vi "Handle Import.vi"(4 "Search Paths":path[](array[path]), 6 "Source .proto":path, 7 "Enumerations in":map{string, T1}(c390), 8 "error in (no error)":errorcluster, 9 "Messages in":map{string, T3}(c390), 10 "Import String":string, 11 "ProtoParser in":refnum<class "ProtoParser.lvclass">) -> (0 "error out":errorcluster, 1 "Messages":map{string, T3}(c390), 3 "ProtoParser out":refnum<class "ProtoParser.lvclass">, 5 "Enumerations":map{string, T1}(c390))   [LabVIEW 2020, in "LV-Protoc.lvlib" / "ProtoParser.lvclass"]
uses:
  ProtoParser.lvclass
  LV-Proto/Message.ctl
  LV-Proto/Field.ctl
  LV-Proto/Type.ctl
  LV-Proto/Proto Type.ctl
  LV-Proto/Enumeration.ctl
  LV-Proto/Enum Value.ctl
  LV-Proto/LV-Proto.lvlib
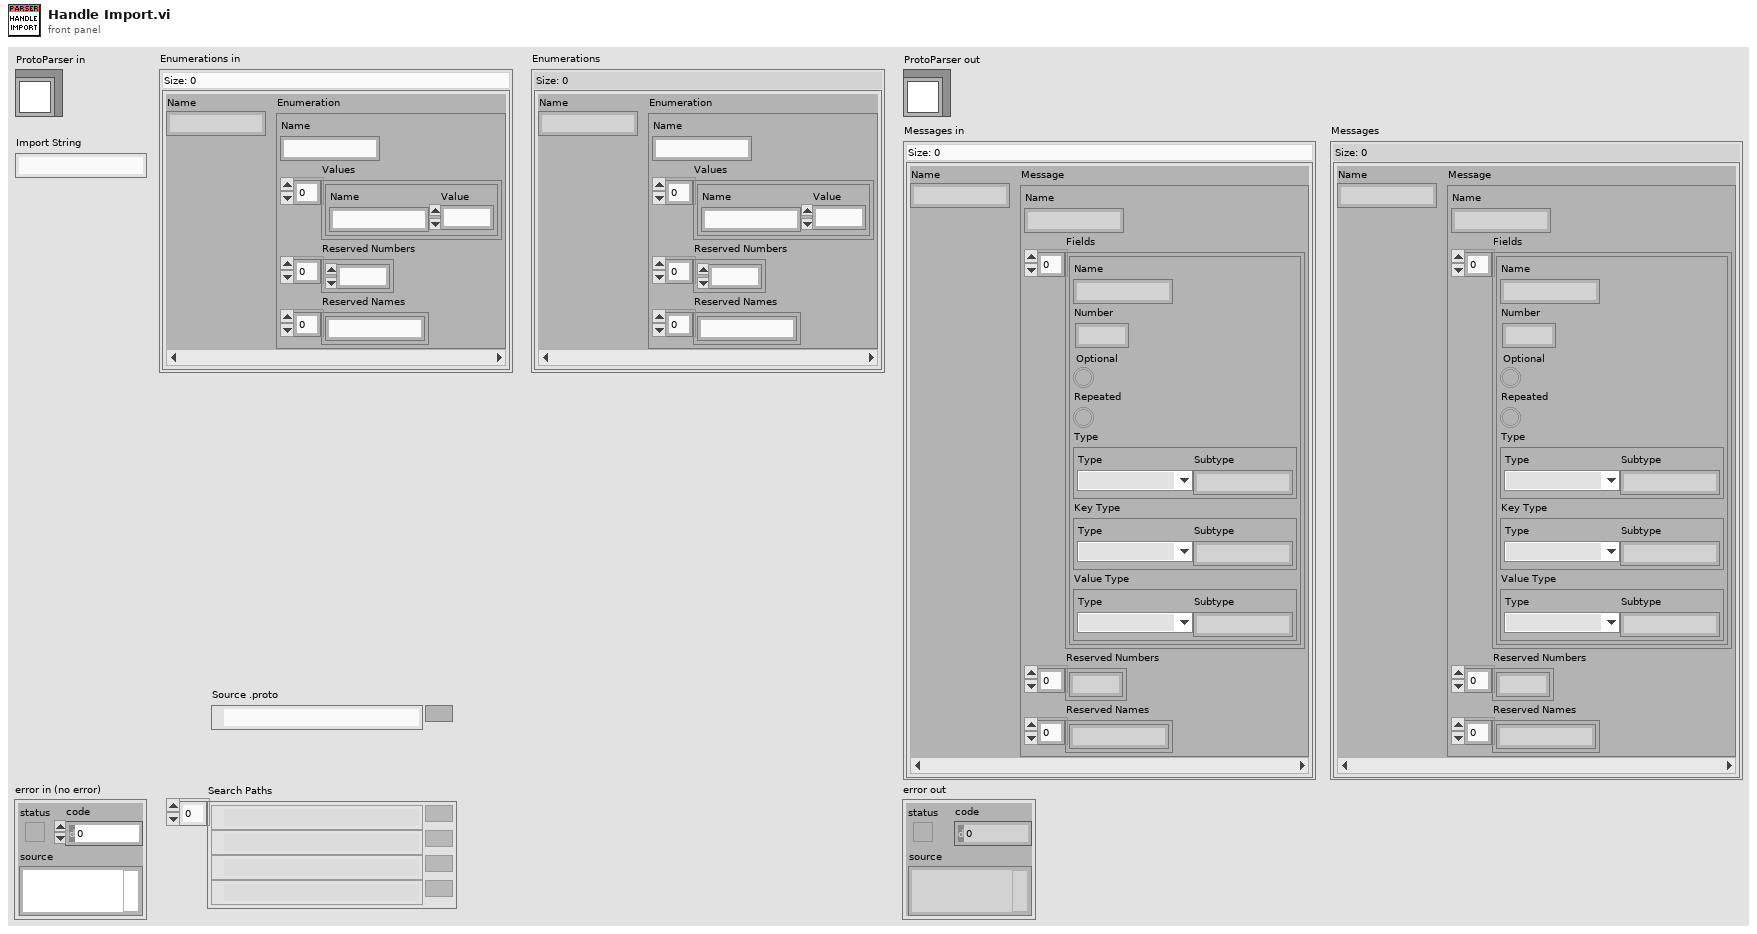
[diagram p1: front panel]
types:
  T1 = typedef "LV-Proto.lvlib/Enumeration.ctl" = cluster{"Name":string, "Values":T2[], "Reserved Numbers":u32[], "Reserved Names":string[]}
  T2 = typedef "LV-Proto.lvlib/Enum Value.ctl" = cluster{"Name":string, "Value":i32}
  T3 = typedef "LV-Proto.lvlib/Message.ctl" = cluster{"Name":string, "Fields":T4[], "Reserved Numbers":u32[], "Reserved Names":string[]}
  T4 = typedef "LV-Proto.lvlib/Field.ctl" = cluster{"Name":string, "Number":u32, "Optional":bool, "Repeated":bool, "Type":T5, "Key Type":T5, "Value Type":T5}
  T5 = typedef "LV-Proto.lvlib/Type.ctl" = cluster{"Type":T6, "Subtype":string}
  T6 = typedef "LV-Proto.lvlib/Proto Type.ctl" = enum16{"UNKNOWN", "double", "float", "int32", "int64", "uint32", "uint64", "sint32", "sint64", "fixed32", "fixed64", "sfixed32", "sfixed64", "bool", "string", "bytes", "enum", "map", "message"}
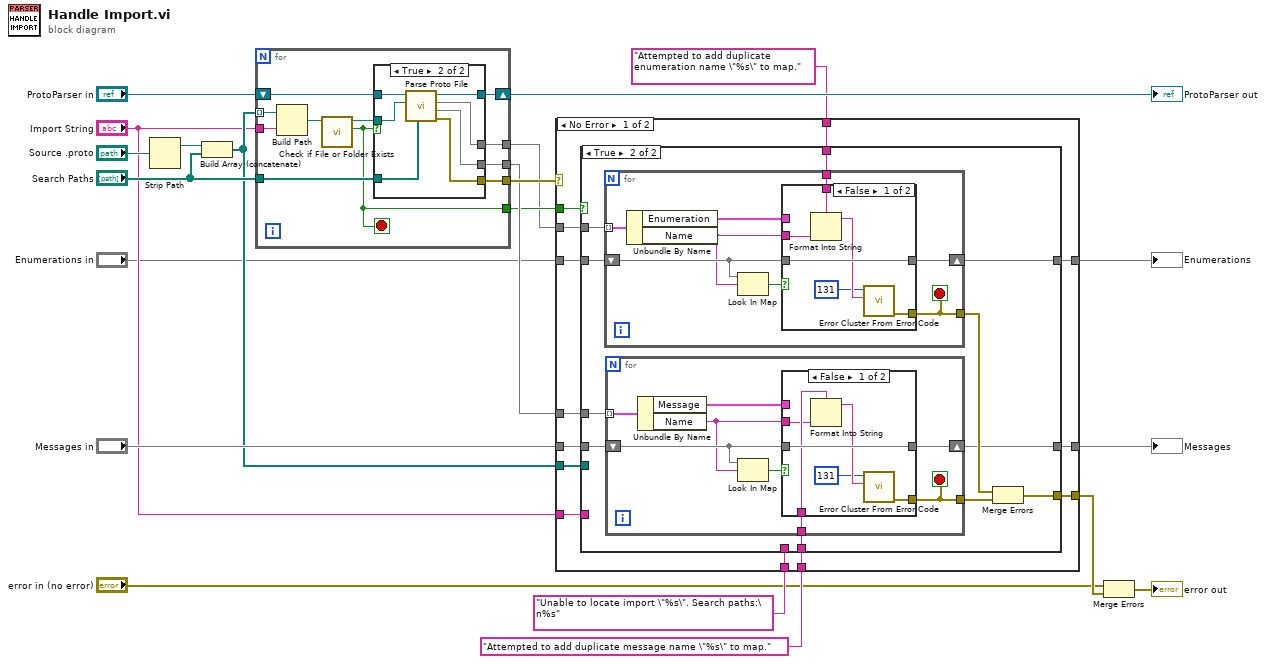
[diagram p0: block diagram]
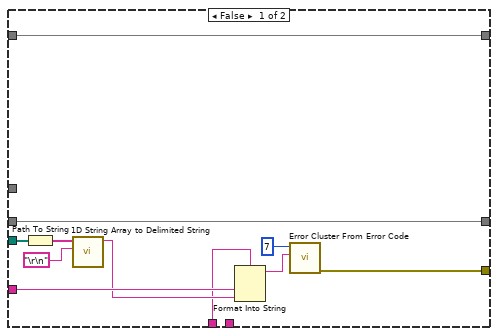
[diagram p2: hidden frame]
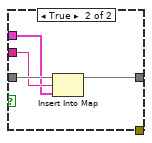
[diagram p3: hidden frame]
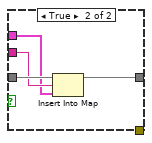
[diagram p4: hidden frame]
diagram:
  n1 = Strip Path(path="Source .proto") -> (stripped path=w19:path)  [unwired: 1 out]
  n2 = Build Array (concatenate)(w19, "Search Paths") -> (w10:path[])
  n3 = for {
    shift-right: [w26] -> w17
    shift-left: "ProtoParser in" -> [w28]
    tunnel: "Import String" -> [w31]
    tunnel: w10 -> [w32] mode=indexing
    tunnel: "Search Paths" -> [w27]
    tunnel: [w25] -> w16
    tunnel: [w24] -> w14
    tunnel: [w23] -> w15
    tunnel: [w22] -> w3
    stop <- w24 stop-if-true
    n4 = Build Path(base path=w32, name or relative path=w31) -> (appended path=w30:path)
    n5 = call <vilib>:"Check if File or Folder Exists.vi"("path"=w30) -> ("file or folder exists?"=w24:bool, "dup path"=w29:path)  [unwired: 8 in, 1 out]
    n6 = case shown="True" w24 {
      tunnel: w29 -> [_ w39]
      tunnel: w28 -> [w33 w40]
      tunnel: w27 -> [_ w38]
      tunnel: [w33 w37] -> w26
      tunnel: [_ w36] -> w25
      tunnel: [_ w35] -> w23
      tunnel: [_ w34] -> w22
      frame False {
      }
      frame True {
        n7 = call "Parse Proto File.vi"("Include Paths (None)"=w38, ".proto Path"=w39, "ProtoParser in"=w40) -> ("error out"=w36:errorcluster, "Messages"=w35:map{string, T3}, "Enumerations"=w34:map{string, T1}, "ProtoParser out"=w37:refnum<class "ProtoParser.lvclass">)  [unwired: 5 in]
      }
    }
  }
  "ProtoParser out" <- w17
  n8 = case shown="No Error" w16 {
    selector: w16 -> [_ w113]
    tunnel: w15 -> [w52 _]
    tunnel: w14 -> [w53 _]
    tunnel: "Messages in" -> [w51 w114]
    tunnel: [w50 w114] -> w12
    tunnel: "Attempted to add duplicate message name \"%s\" to map." -> [w49 _]
    tunnel: [w48 w113] -> w7
    tunnel: w10 -> [w47 _]
    tunnel: "Import String" -> [w46 _]
    tunnel: "Unable to locate import \"%s\". Search paths:\n%s" -> [w45 _]
    tunnel: "Enumerations in" -> [w44 w112]
    tunnel: w3 -> [w43 _]
    tunnel: [w42 w112] -> w2
    tunnel: "Attempted to add duplicate enumeration name \"%s\" to map." -> [w41 _]
    frame No Error {
      n9 = case shown="True" w53 {
        tunnel: w52 -> [_ w73]
        tunnel: w51 -> [w64 w74]
        tunnel: [w64 w72] -> w50
        tunnel: w49 -> [_ w71]
        tunnel: [w58 w69] -> w48
        tunnel: w47 -> [w63 _]
        tunnel: w46 -> [w60 _]
        tunnel: w45 -> [w55 _]
        tunnel: w44 -> [w54 w67]
        tunnel: w43 -> [_ w68]
        tunnel: [w54 w66] -> w42
        tunnel: w41 -> [_ w65]
        frame False {
          n10 = Path To String(path=w63) -> (string=w62:string[])
          n11 = call <vilib>:"1D String Array to Delimited String.vi"("delimiter"="\r\n", "string array"=w62) -> ("delimited string"=w59:string)  [unwired: 9 in]
          n12 = Format Into String(format string=w55, w60, w59) -> (resulting string=w56:string)  [unwired: 2 in, 1 out]
          n13 = call <vilib>:"Error Cluster From Error Code.vi"("error message (\"\")"=w56, "error code (0)"=7) -> ("error out"=w58:errorcluster)  [unwired: 7 in]
        }
        frame True {
          n14 = for {
            shift-right: [w78] -> w66
            shift-left: w67 -> [w81]
            tunnel: w68 -> [w83] mode=indexing
            tunnel: [w77] -> w75
            tunnel: w65 -> [w76]
            stop <- w77 stop-if-true
            n15 = Unbundle By Name(w83) -> ("Enumeration"=w80:T1, "Name"=w79:string)
            n16 = Look In Map(map=w81, key=w79) -> (key not found?=w82:bool)  [unwired: 1 in, 1 out]
            n17 = case shown="False" w82 {
              tunnel: w81 -> [w89 w93]
              tunnel: w80 -> [_ w91]
              tunnel: w79 -> [w88 w92]
              tunnel: [w89 w90] -> w78
              tunnel: [w85 _] -> w77
              tunnel: w76 -> [w84 _]
              frame False {
                n18 = Format Into String(format string=w84, w88) -> (resulting string=w87:string)  [unwired: 2 in, 1 out]
                n19 = call <vilib>:"Error Cluster From Error Code.vi"("error message (\"\")"=w87, "error code (0)"=131) -> ("error out"=w85:errorcluster)  [unwired: 7 in]
              }
              frame True {
                n20 = Insert Into Map(map in=w93, key=w92, value=w91) -> (map out=w90:map{string, T1})  [unwired: 2 out]
              }
            }
          }
          n21 = for {
            shift-right: [w96] -> w72
            shift-left: w74 -> [w99]
            tunnel: w73 -> [w101] mode=indexing
            tunnel: w71 -> [w95]
            tunnel: [w94] -> w70
            stop <- w94 stop-if-true
            n22 = Unbundle By Name(w101) -> ("Message"=w98:T3, "Name"=w97:string)
            n23 = Look In Map(map=w99, key=w97) -> (key not found?=w100:bool)  [unwired: 1 in, 1 out]
            n24 = case shown="False" w100 {
              tunnel: w99 -> [w107 w111]
              tunnel: w98 -> [_ w109]
              tunnel: w97 -> [w105 w110]
              tunnel: [w107 w108] -> w96
              tunnel: w95 -> [w106 _]
              tunnel: [w102 _] -> w94
              frame False {
                n25 = Format Into String(format string=w106, w105) -> (resulting string=w104:string)  [unwired: 2 in, 1 out]
                n26 = call <vilib>:"Error Cluster From Error Code.vi"("error message (\"\")"=w104, "error code (0)"=131) -> ("error out"=w102:errorcluster)  [unwired: 7 in]
              }
              frame True {
                n27 = Insert Into Map(map in=w111, key=w110, value=w109) -> (map out=w108:map{string, T3})  [unwired: 2 out]
              }
            }
          }
          n28 = Merge Errors(w75, w70) -> (w69:errorcluster)
        }
      }
    }
    frame Error {
    }
  }
  "Messages" <- w12
  "Enumerations" <- w2
  n29 = Merge Errors("error in (no error)", w7) -> (→"error out":errorcluster)
